vi "normalise_T1.vi"(10 "normalise":bool=TRUE, 11 "T1_curve_in":cluster{"dark_time_us":dbl[], "PL_signal":dbl[]}) -> (3 "T1_curve_out":cluster{"dark_time_us":dbl[], "PL_signal":dbl[]})   [LabVIEW 2014]
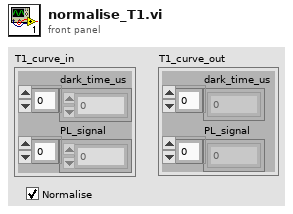
[diagram p1: front panel]
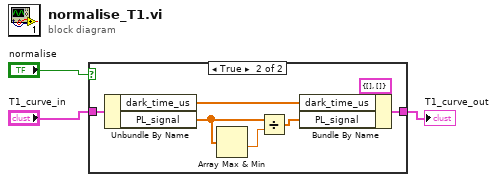
[diagram p0: block diagram]
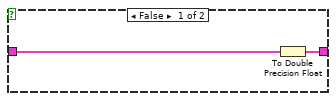
[diagram p2: hidden frame]
diagram:
  n1 = case shown="True" "normalise" {
    tunnel: "T1_curve_in" -> [w5 w11]
    tunnel: [w4 w8] -> w3
    frame False {
      n2 = To Double Precision Float(number=w5) -> (double precision float=w4:cluster{"dark_time_us":dbl[], "PL_signal":dbl[]})
    }
    frame True {
      n3 = Unbundle By Name(w11) -> ("dark_time_us"=w10:dbl[], "PL_signal"=w6:dbl[])
      n4 = Array Max & Min(array=w6) -> (min value=w12:dbl)  [unwired: 3 out]
      n5 = Divide(x=w6, y=w12) -> (x/y=w9:dbl[])
      n6 = Bundle By Name(cluster=cluster{"dark_time_us":dbl[], "PL_signal":dbl[]} {"dark_time_us"=[], "PL_signal"=[]} ("T1 curve"), "dark_time_us"=w10, "PL_signal"=w9) -> (w8:cluster{"dark_time_us":dbl[], "PL_signal":dbl[]})
    }
  }
  "T1_curve_out" <- w3
